vi "MTIF_Write_2D2B.vi"(6 "Record?":bool, 7 "Byte Order":T1(ring)=enum."little-endian", 8 "error in (no error)":errorcluster, 9 "Image Data Array":u16[][](array[numeric]), 10 "Start Sequence? In":bool, 11 "Byte Stream File In":refnum<file>) -> (0 "error out":errorcluster, 2 "Start Sequence? Out":bool, 3 "Byte Stream File Out":refnum<file>)   [LabVIEW 2014]
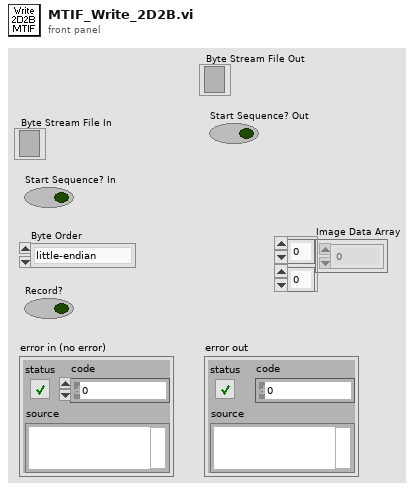
[diagram p1: front panel]
types:
  T1 = enum16{"big-endian, network order", "native, host order", "little-endian"}
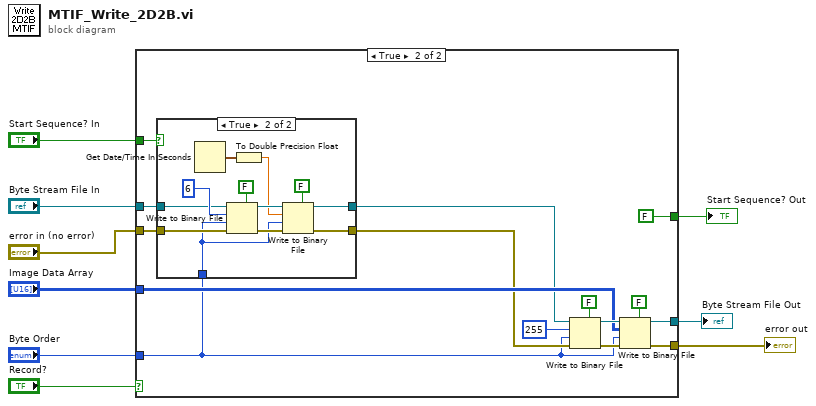
[diagram p0: block diagram]
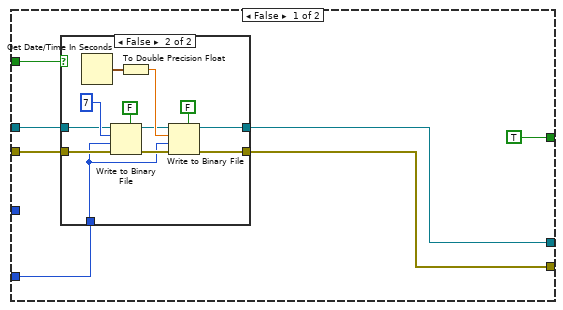
[diagram p2: hidden frame]
diagram:
  n1 = case shown="True" "Record?" {
    tunnel: "Image Data Array" -> [_ w38]
    tunnel: "Byte Stream File In" -> [w15 w33]
    tunnel: [w11 w44] -> w3
    tunnel: "Byte Order" -> [w16 w34]
    tunnel: "error in (no error)" -> [w14 w35]
    tunnel: [w10 w43] -> w7
    tunnel: "Start Sequence? In" -> [w13 w37]
    tunnel: [TRUE ("Record?") FALSE ("Record?")] -> w9
    frame False {
      n2 = case shown="False" w13 {
        tunnel: [w18 w19] -> w10
        tunnel: w14 -> [w18 w28]
        tunnel: w16 -> [_ w21]
        tunnel: w15 -> [w17 w27]
        tunnel: [w17 w20] -> w11
        frame True {
        }
        frame False {
          n3 = Get Date/Time In Seconds() -> (seconds since 1Jan1904=w25:timestamp)
          n4 = Write to Binary File(file (use dialog)=w27, data=u8 7, error in=w28, 5:FALSE ("prepend array or string size? (T)"), 9:w21) -> (refnum out=w23:refnum<file>, error out=w22:errorcluster)  [unwired: 1 in, 1 out]
          n5 = To Double Precision Float(number=w25) -> (double precision float=w24:dbl)
          n6 = Write to Binary File(file (use dialog)=w23, data=w24, error in=w22, 5:FALSE ("prepend array or string size? (T)"), 9:w21) -> (refnum out=w20:refnum<file>, error out=w19:errorcluster)  [unwired: 1 in, 1 out]
        }
      }
    }
    frame True {
      n7 = case shown="True" w37 {
        tunnel: [w47 w49] -> w36
        tunnel: w35 -> [w47 w57]
        tunnel: w34 -> [_ w50]
        tunnel: w33 -> [w46 w56]
        tunnel: [w46 w48] -> w32
        frame False {
        }
        frame True {
          n8 = Get Date/Time In Seconds() -> (seconds since 1Jan1904=w52:timestamp)
          n9 = Write to Binary File(file (use dialog)=w56, data=u8 6, error in=w57, 5:FALSE ("prepend array or string size? (T)"), 9:w50) -> (refnum out=w54:refnum<file>, error out=w53:errorcluster)  [unwired: 1 in, 1 out]
          n10 = To Double Precision Float(number=w52) -> (double precision float=w51:dbl)
          n11 = Write to Binary File(file (use dialog)=w54, data=w51, error in=w53, 5:FALSE ("prepend array or string size? (T)"), 9:w50) -> (refnum out=w48:refnum<file>, error out=w49:errorcluster)  [unwired: 1 in, 1 out]
        }
      }
      n12 = Write to Binary File(file (use dialog)=w32, data=u8 255, error in=w36, 5:FALSE ("prepend array or string size? (T)"), 9:w34) -> (refnum out=w40:refnum<file>, error out=w39:errorcluster)  [unwired: 1 in, 1 out]
      n13 = Write to Binary File(file (use dialog)=w40, data=w38, error in=w39, 5:FALSE ("prepend array or string size? (T)"), 9:w34) -> (refnum out=w44:refnum<file>, error out=w43:errorcluster)  [unwired: 1 in, 1 out]
    }
  }
  "Start Sequence? Out" <- w9
  "error out" <- w7
  "Byte Stream File Out" <- w3
